vi "Differentiate 18bfxp1s.vi"(1 "Output":fxp<+/-,18,1> format="%.18g") -> (0 "Numeric":fxp<+/-,18,1> format="%.18g")   [LabVIEW 2009]
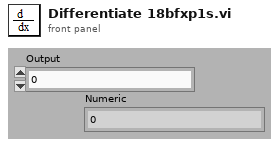
[diagram p1: front panel]
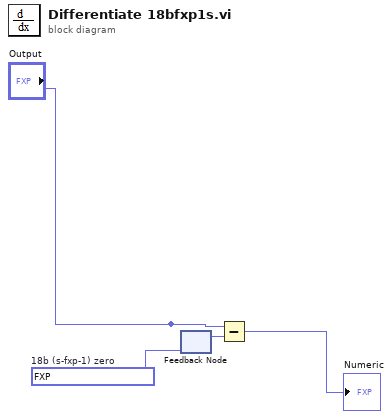
[diagram p0: block diagram]
diagram:
  w3 = fxp<+/-,18,1> 0.0  # 18b (s-fxp-1) zero
  n1 = feedback #1(w3) -> (w2:fxp<+/-,18,1>)
  n2 = Subtract(x="Output", y=w2) -> (x-y=→"Numeric":fxp<+/-,18,1>)
